vi "angle-statstics-test.vi"() -> (3 "All Passed":bool)   [LabVIEW 2019]
uses:
  <vilib>/Analysis/Matrix/Datatypes/RealMatrix.ctl
  <vilib>/Rock Robotics/WPI/ThirdParty/JAS_Junk/TrajLib/MatBuilder_Create.vi
  <vilib>/Rock Robotics/WPI/ThirdParty/JAS_Junk/TrajLib/Trajectory_Library.lvlib
  <vilib>/Analysis/Matrix/NI_Matrix.lvlib
panel:
  out "Passed 3A":bool
  out "Passed 3":bool
  out "Passed 2A":bool
  out "Passed 2":bool
  out "Passed 1A":bool
  out "Passed 1":bool
  out "Error1":bool
  out "Error 3A":bool
  out "Result 3A":T1
  out "Result 3":T1
  out "Error 2A":bool
  out "Result 2A":T1
  out "Result 2":T1
  out "Error 1A":bool
  out "Result 1A":T1
  out "Result 1":T1
  # "MEAN"
  # "RESIDUAL (MINUS)"
  # "ADD"
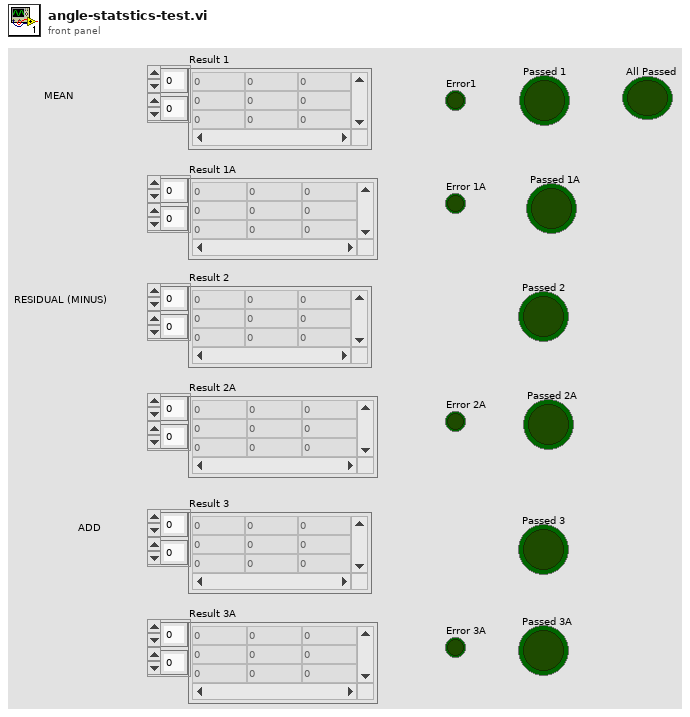
[diagram p1: front panel]
types:
  T1 = typedef "NI_Matrix.lvlib/RealMatrix.ctl" = dbl[][]
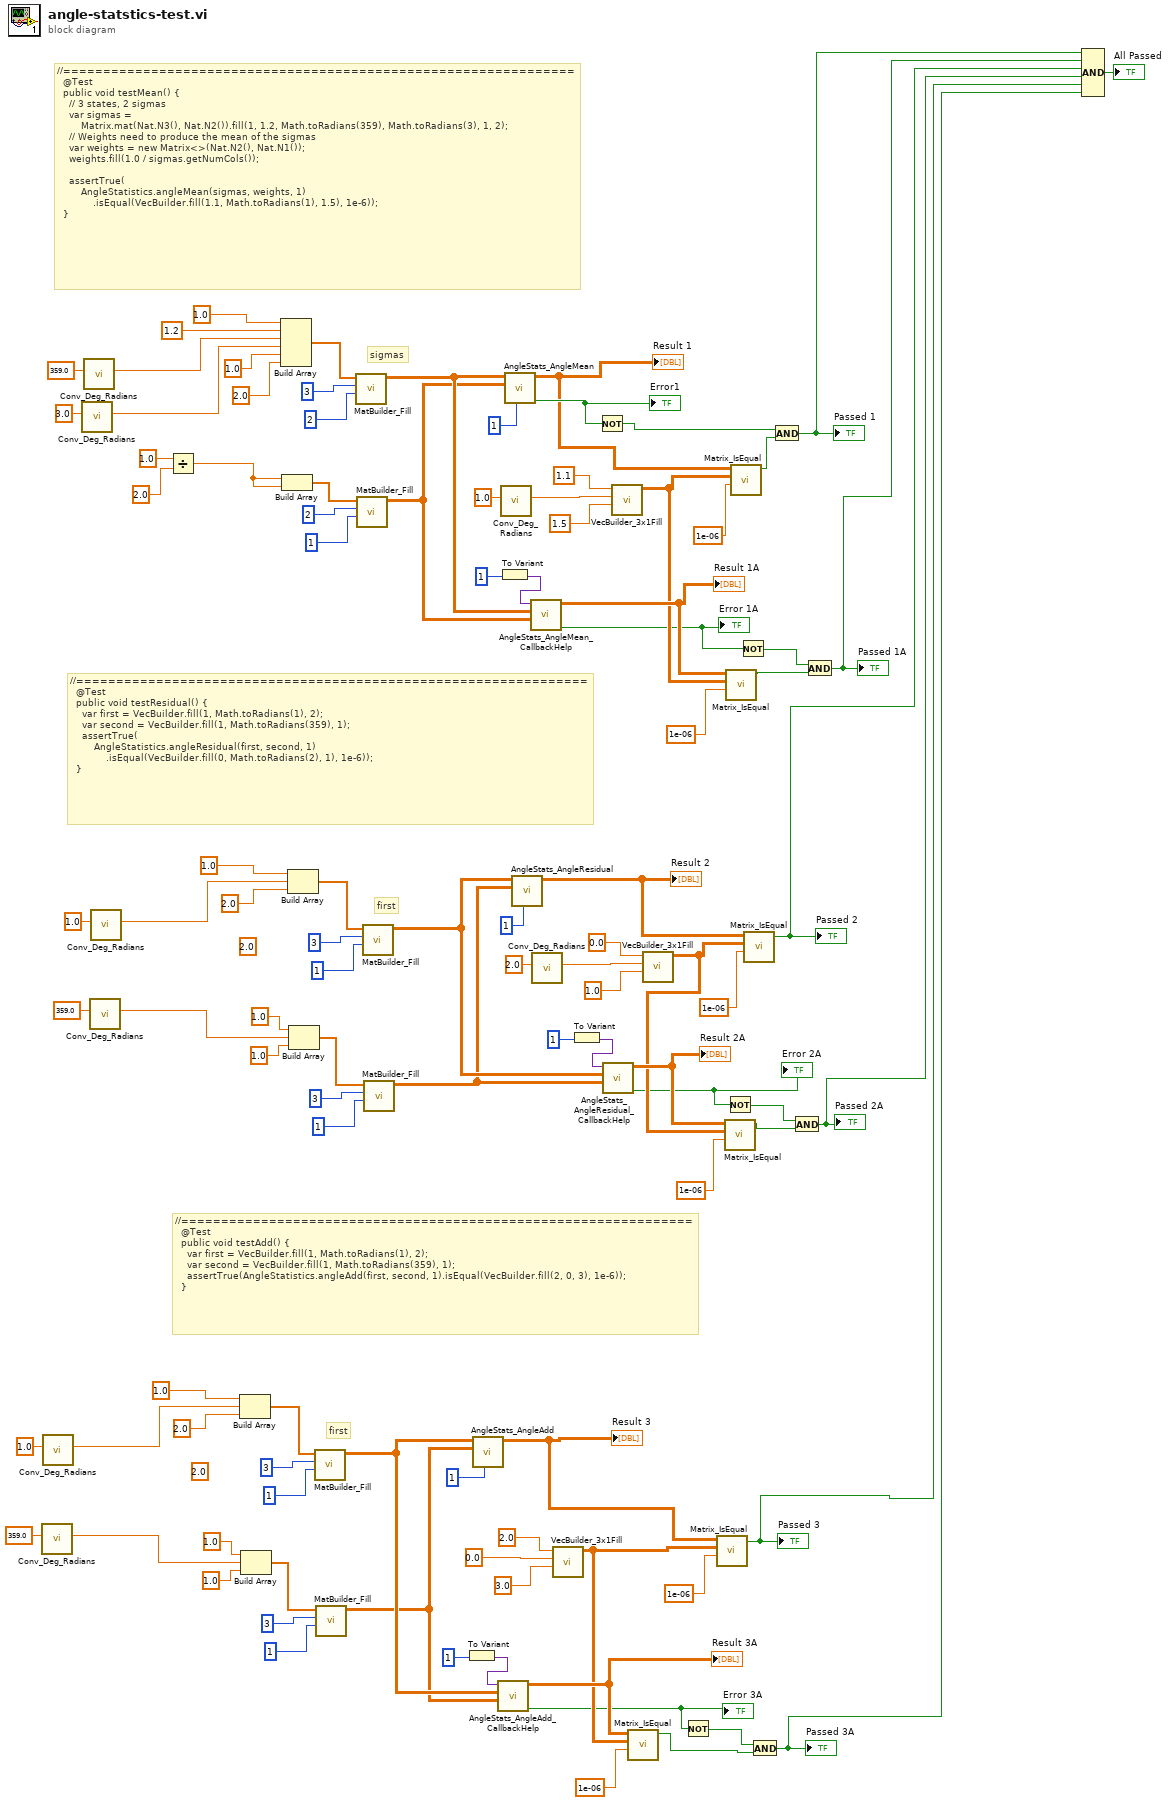
[diagram p0: block diagram]
diagram:
  (unwired) 2.0 ("element")
  (unwired) 2.0 ("element")
  # "first"
  # "//================================================================\n  @Test\n  public void testAdd() {\n    var first = VecBuilder.fill(1, Math.toRadians(1), 2);\n    var second = VecBuilder.fill(1, Math.toRadians(359), 1);\n    assertTrue(AngleStatistics.angleAdd(first, second, 1).isEqual(VecBuilder.fill(2, 0, 3), 1e-6));\n  }"
  # "first"
  # "//================================================================\n  @Test\n  public void testResidual() {\n    var first = VecBuilder.fill(1, Math.toRadians(1), 2);\n    var second = VecBuilder.fill(1, Math.toRadians(359), 1);\n    assertTrue(\n        AngleStatistics.angleResidual(first, second, 1)\n            .isEqual(VecBuilder.fill(0, Math.toRadians(2), 1), 1e-6));\n  }"
  # "sigmas"
  # "//================================================================\n  @Test\n  public void testMean() {\n    // 3 states, 2 sigmas\n    var sigmas =\n        Matrix.mat(Nat.N3(), Nat.N2()).fill(1, 1.2, Math.toRadians(359), Math.toRadians(3), 1, 2);\n    // Weights need to produce the mean of the sigmas\n    var weights = new Matrix<>(Nat.N2(), Nat.N1());\n    weights.fill(1.0 / sigmas.getNumCols());\n\n    assertTrue(\n        AngleStatistics.angleMean(sigmas, weights, 1)\n            .isEqual(VecBuilder.fill(1.1, Math.toRadians(1), 1.5), 1e-6));\n  }"
  n1 = call <vilib>:"Conv_Deg_Radians.vi"("Degress"=359.0) -> ("Radians"=w46:dbl)  [unwired: 10 in]
  n2 = call <vilib>:"Conv_Deg_Radians.vi"("Degress"=1.0) -> ("Radians"=w49:dbl)  [unwired: 10 in]
  n3 = call <vilib>:"Conv_Deg_Radians.vi"("Degress"=3.0) -> ("Radians"=w97:dbl)  [unwired: 10 in]
  n4 = call <vilib>:"Conv_Deg_Radians.vi"("Degress"=359.0) -> ("Radians"=w98:dbl)  [unwired: 10 in]
  n5 = call <vilib>:"Conv_Deg_Radians.vi"("Degress"=359.0) -> ("Radians"=w65:dbl)  [unwired: 10 in]
  n6 = call <vilib>:"Conv_Deg_Radians.vi"("Degress"=1.0) -> ("Radians"=w68:dbl)  [unwired: 10 in]
  n7 = Divide(x=1.0, y=2.0) -> (x/y=w90:dbl)
  n8 = Build Array(1.0 ("element"), w49, 2.0 ("element")) -> (w61:dbl[])
  n9 = Build Array(1.0 ("element"), w46, 1.0 ("element")) -> (w55:dbl[])
  n10 = Build Array(1.0 ("element"), 1.2 ("element"), w98, w97, 1.0 ("element"), 2.0 ("element")) -> (w103:dbl[])
  n11 = Build Array(w90, w90) -> (w89:dbl[])
  n12 = Build Array(1.0 ("element"), w68, 2.0 ("element")) -> (w80:dbl[])
  n13 = Build Array(1.0 ("element"), w65, 1.0 ("element")) -> (w74:dbl[])
  n14 = call <vilib>:"MatBuilder_Fill.vi"("Columns"=1, "Rows"=3, "Value List"=w61) -> ("output matrix"=w53:T1)  [unwired: 8 in]
  n15 = call <vilib>:"MatBuilder_Fill.vi"("Columns"=1, "Rows"=3, "Value List"=w55) -> ("output matrix"=w52:T1)  [unwired: 8 in]
  n16 = call <vilib>:"MatBuilder_Fill.vi"("Columns"=2, "Rows"=3, "Value List"=w103) -> ("output matrix"=w87:T1)  [unwired: 8 in]
  n17 = call <vilib>:"MatBuilder_Fill.vi"("Columns"=1, "Rows"=2, "Value List"=w89) -> ("output matrix"=w86:T1)  [unwired: 8 in]
  n18 = call <vilib>:"MatBuilder_Fill.vi"("Columns"=1, "Rows"=3, "Value List"=w80) -> ("output matrix"=w72:T1)  [unwired: 8 in]
  n19 = call <vilib>:"MatBuilder_Fill.vi"("Columns"=1, "Rows"=3, "Value List"=w74) -> ("output matrix"=w71:T1)  [unwired: 8 in]
  n20 = To Variant(anything=1) -> (Variant=w50:variant)
  n21 = call <vilib>:"AngleStats_AngleAdd.vi"("Row"=1, "B"=w52, "A"=w53) -> ("Result"=w15:T1)  [unwired: 8 in]
  "Result 3" <- w15
  n22 = call <vilib>:"AngleStats_AngleAdd_CallbackHelp.vi"("B"=w52, "A"=w53, "ExtraPassedData"=w50) -> ("Error"=w8:bool, "Result"=w12:T1)  [unwired: 7 in]
  "Result 3A" <- w12
  "Error 3A" <- w8
  n23 = To Variant(anything=1) -> (Variant=w83:variant)
  n24 = call <vilib>:"Conv_Deg_Radians.vi"("Degress"=1.0) -> ("Radians"=w43:dbl)  [unwired: 10 in]
  n25 = call <vilib>:"AngleStats_AngleMean.vi"("Row"=1, "Wm"=w86, "Sigmas"=w87) -> ("Error"=w40:bool, "Result"=w38:T1)  [unwired: 7 in]
  "Result 1" <- w38
  "Error1" <- w40
  n26 = call <vilib>:"AngleStats_AngleResidual.vi"("Row"=1, "B"=w71, "A"=w72) -> ("Result"=w25:T1)  [unwired: 8 in]
  "Result 2" <- w25
  n27 = call <vilib>:"AngleStats_AngleMean_CallbackHelp.vi"("B"=w86, "A"=w87, "ExtraPassedData"=w83) -> ("Error"=w33:bool, "Result"=w35:T1)  [unwired: 7 in]
  "Result 1A" <- w35
  "Error 1A" <- w33
  n28 = call <vilib>:"Conv_Deg_Radians.vi"("Degress"=2.0) -> ("Radians"=w28:dbl)  [unwired: 10 in]
  n29 = call <vilib>:"VecBuilder_3x1Fill.vi"("R2"=3.0, "R1"=0.0 ("Degress"), "R0"=2.0) -> ("output matrix"=w11:T1)  [unwired: 8 in]
  n30 = To Variant(anything=1) -> (Variant=w69:variant)
  n31 = Not(x=w40) -> (.not. x?=w39:bool)
  n32 = call <vilib>:"AngleStats_AngleResidual_CallbackHelp.vi"("B"=w71, "A"=w72, "ExtraPassedData"=w69) -> ("Error"=w20:bool, "Result"=w23:T1)  [unwired: 7 in]
  "Result 2A" <- w23
  "Error 2A" <- w20
  n33 = call <vilib>:"VecBuilder_3x1Fill.vi"("R2"=1.5, "R1"=w43, "R0"=1.1) -> ("output matrix"=w34:T1)  [unwired: 8 in]
  n34 = call <vilib>:"Matrix_IsEqual.vi"("Tolerance"=1e-06, "other"=w11, "input matrix"=w12) -> ("Equal"=w9:bool)  [unwired: 8 in]
  n35 = call <vilib>:"VecBuilder_3x1Fill.vi"("R2"=1.0, "R1"=w28, "R0"=0.0) -> ("output matrix"=w22:T1)  [unwired: 8 in]
  n36 = Not(x=w8) -> (.not. x?=w10:bool)
  n37 = call <vilib>:"Matrix_IsEqual.vi"("Tolerance"=1e-06, "other"=w11, "input matrix"=w15) -> ("Equal"=w3:bool)  [unwired: 8 in]
  "Passed 3" <- w3
  n38 = Not(x=w20) -> (.not. x?=w21:bool)
  n39 = call <vilib>:"Matrix_IsEqual.vi"("Tolerance"=1e-06, "other"=w22, "input matrix"=w23) -> ("Equal"=w19:bool)  [unwired: 8 in]
  n40 = call <vilib>:"Matrix_IsEqual.vi"("Tolerance"=1e-06, "other"=w34, "input matrix"=w35) -> ("Equal"=w32:bool)  [unwired: 8 in]
  n41 = call <vilib>:"Matrix_IsEqual.vi"("Tolerance"=1e-06, "other"=w34, "input matrix"=w38) -> ("Equal"=w37:bool)  [unwired: 8 in]
  n42 = Not(x=w33) -> (.not. x?=w31:bool)
  n43 = call <vilib>:"Matrix_IsEqual.vi"("Tolerance"=1e-06, "other"=w22, "input matrix"=w25) -> ("Equal"=w5:bool)  [unwired: 8 in]
  "Passed 2" <- w5
  n44 = And(x=w10, y=w9) -> (x .and. y?=w2:bool)
  "Passed 3A" <- w2
  n45 = And(x=w39, y=w37) -> (x .and. y?=w7:bool)
  "Passed 1" <- w7
  n46 = And(x=w21, y=w19) -> (x .and. y?=w4:bool)
  "Passed 2A" <- w4
  n47 = And(x=w31, y=w32) -> (x .and. y?=w6:bool)
  "Passed 1A" <- w6
  n48 = Compound Arithmetic op=AND(w7, w6, w5, w4, w3, w2) -> (→"All Passed":bool)
